vi "main.vi"() -> ()   [LabVIEW 2023]
uses:
  #typedef_States.ctl
  #typedef_DeviceInfo.ctl
panel:
  out "Centrifugation":bool
  in  "Start":bool
  in  "Lid 0pen":bool
  in  "Centrifugation":bool
  out "Lid Open":bool
  out "Blood Cedimentation (OB)":bool
  out "Hormones":bool
  out "Cancer Markers":bool
  out "Blood Cell Count":bool
  out "Centrifugation":bool
  out "Power ON":bool
  in  "Mode":i32(knob)=2 scale=0.0..4.0
  in  "Stop":bool
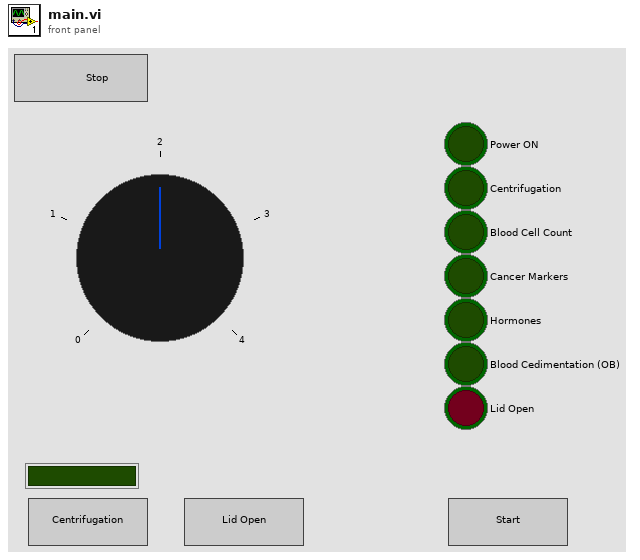
[diagram p1: front panel]
types:
  T1 = typedef "#typedef_States.ctl" = enum16{"Initialize", "Idle", "TestInit", "Test", "LidOpen", "Wait", "TurnOff", "Exit"}
  T2 = enum8{"Enabled", "Disabled", "Disabled and Grayed Out"}
  T3 = typedef "#typedef_DeviceInfo.ctl" = cluster{"Mode":enum16{"Fast Test", "Basic Test", "Power Off", "Full Test", "High Quality Test"}, "Time":cluster{"Centrifugation":i32, "Blood Cell Count":i32, "Cancer Makers":i32, "Hormones":i32, "Blood Cedimentation":i32}, "LidOpenTime":dbl, "Current Time":timestamp, "TestState":i32, "TimeToWait":i32}
  T4 = enum16{"Fast Test", "Basic Test", "Power Off", "Full Test", "High Quality Test"}
  T5 = cluster{"Centrifugation":i32, "Blood Cell Count":i32, "Cancer Makers":i32, "Hormones":i32, "Blood Cedimentation":i32}
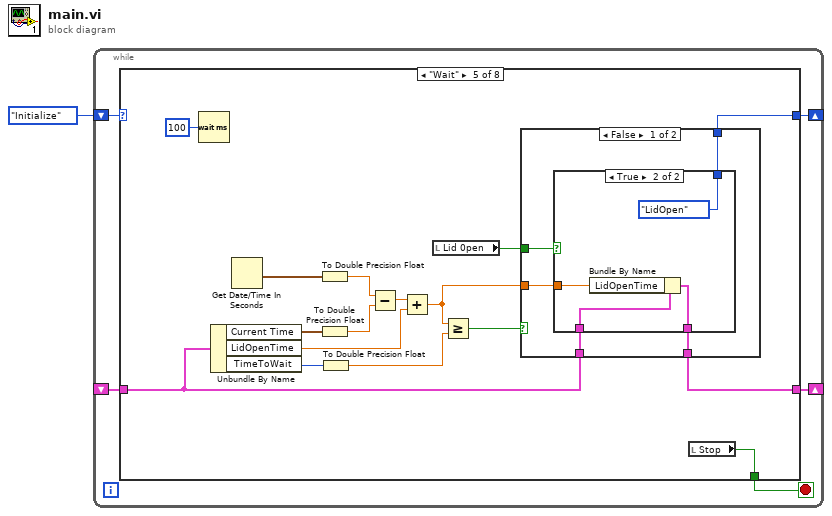
[diagram p0: block diagram]
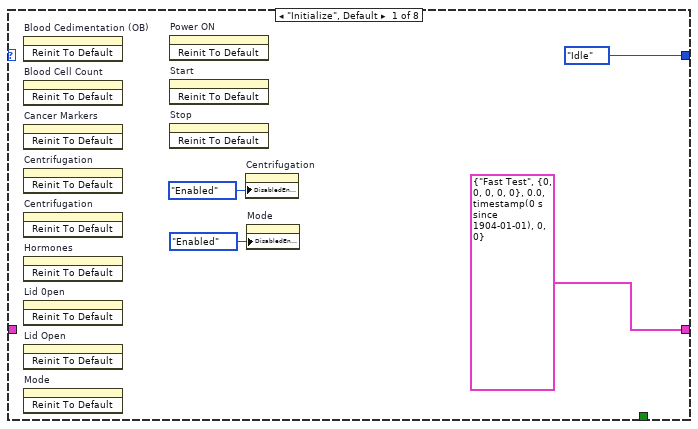
[diagram p2: hidden frame]
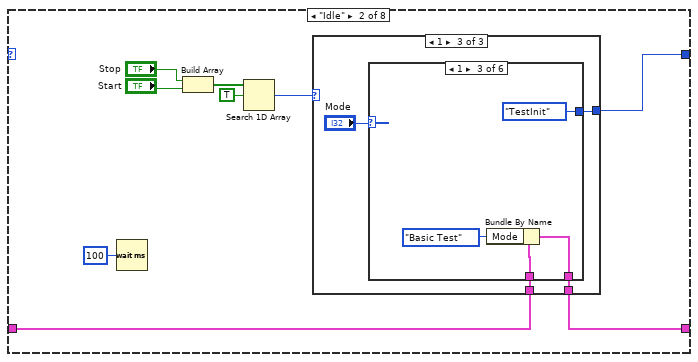
[diagram p3: hidden frame]
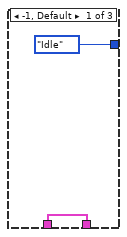
[diagram p4: hidden frame]
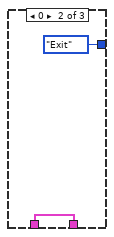
[diagram p5: hidden frame]
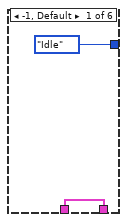
[diagram p6: hidden frame]
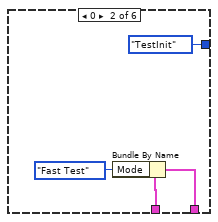
[diagram p7: hidden frame]
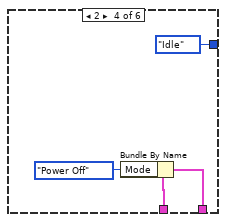
[diagram p8: hidden frame]
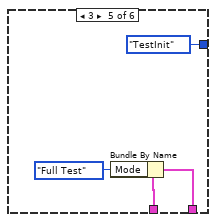
[diagram p9: hidden frame]
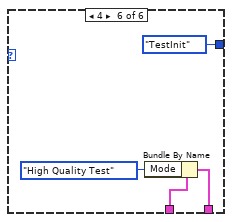
[diagram p10: hidden frame]
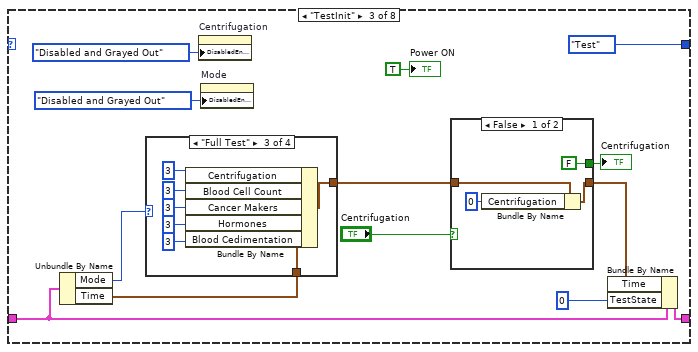
[diagram p11: hidden frame]
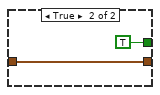
[diagram p12: hidden frame]
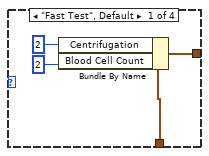
[diagram p13: hidden frame]
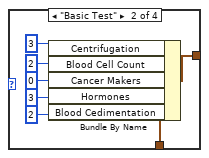
[diagram p14: hidden frame]
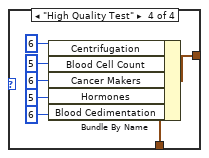
[diagram p15: hidden frame]
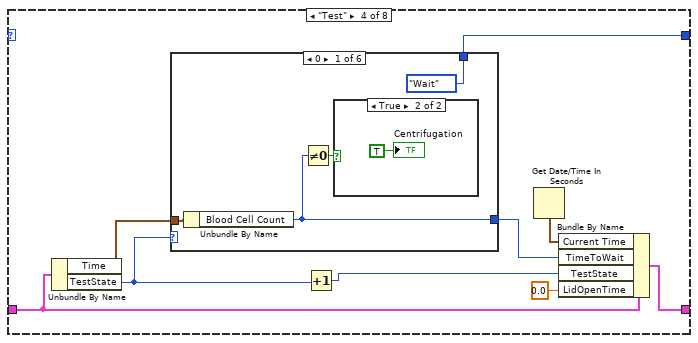
[diagram p16: hidden frame]
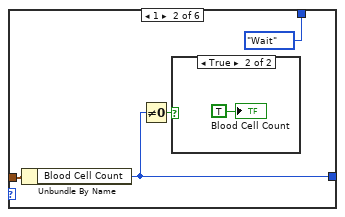
[diagram p18: hidden frame]
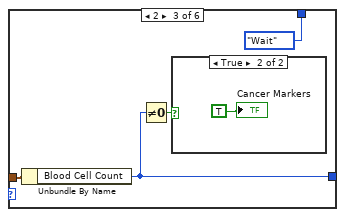
[diagram p20: hidden frame]
diagram:
  n1 = while {
    shift-right: [w5] -> _
    shift-left: #typedef_States."Initialize" ("States") -> [w6]
    shift-right: [w4] -> _
    shift-left: _ -> [w3]
    stop <- w2 stop-if-true
    n2 = case shown="\"Wait\"" w6 {
      tunnel: [#typedef_States."Idle" ("States") w14 #typedef_States."Test" ("States") w98 w133 #typedef_States."Test" ("States") w165 #typedef_States."Exit" ("States")] -> w5
      tunnel: [T3 {"Mode"=enum."Fast Test", "Time"={"Centrifugation"=0, "Blood Cell Count"=0, "Cancer Makers"=0, "Hormones"=0, "Blood Cedimentation"=0}, "LidOpenTime"=0.0, "Current Time"=timestamp(0 s since 1904-01-01), "TestState"=0, "TimeToWait"=0} ("DeviceInfo") w12 w56 w100 w134 w160 w163 w174] -> w4
      tunnel: w3 -> [_ w13 w57 w101 w135 w160 w164 w174]
      tunnel: [_ _ _ _ w140 _ _ TRUE] -> w2
      frame "Initialize", Default {
        n3 = invoke on="Blood Cedimentation (OB)" class="Bool (strict)" method="Reinit To Default"() -> ()  [unwired: 3 in, 3 out]
        n4 = invoke on="Blood Cell Count" class="Bool (strict)" method="Reinit To Default"() -> ()  [unwired: 3 in, 3 out]
        n5 = invoke on="Cancer Markers" class="Bool (strict)" method="Reinit To Default"() -> ()  [unwired: 3 in, 3 out]
        n6 = invoke on="Centrifugation" class="Bool (strict)" method="Reinit To Default"() -> ()  [unwired: 3 in, 3 out]
        n7 = invoke on="Centrifugation" class="Bool (strict)" method="Reinit To Default"() -> ()  [unwired: 3 in, 3 out]
        n8 = invoke on="Hormones" class="Bool (strict)" method="Reinit To Default"() -> ()  [unwired: 3 in, 3 out]
        n9 = invoke on="Lid 0pen" class="Bool (strict)" method="Reinit To Default"() -> ()  [unwired: 3 in, 3 out]
        n10 = invoke on="Lid Open" class="Bool (strict)" method="Reinit To Default"() -> ()  [unwired: 3 in, 3 out]
        n11 = invoke on="Mode" class="Knob (strict)" method="Reinit To Default"() -> ()  [unwired: 3 in, 3 out]
        n12 = invoke on="Power ON" class="Bool (strict)" method="Reinit To Default"() -> ()  [unwired: 3 in, 3 out]
        n13 = invoke on="Start" class="Bool" method="Reinit To Default"() -> ()  [unwired: 3 in, 3 out]
        n14 = invoke on="Stop" class="Bool (strict)" method="Reinit To Default"() -> ()  [unwired: 3 in, 3 out]
        n15 = property on="Centrifugation" class="Bool (strict)"("DisabledEnum"=T2."Enabled" ("Disabled")) -> ()  [unwired: 2 in, 2 out]
        n16 = property on="Mode" class="Knob (strict)"("DisabledEnum"=T2."Enabled" ("Disabled")) -> ()  [unwired: 2 in, 2 out]
      }
      frame "Idle" {
        n17 = Wait (ms)(milliseconds to wait=u32 100) -> ()  [unwired: 1 out]
        n18 = Build Array("Stop", "Start") -> (w19:bool[])
        n19 = Search 1D Array(1D array=w19, element=TRUE) -> (index of element=w15:i32)  [unwired: 1 in]
        n20 = case shown="1" w15 {
          tunnel: [#typedef_States."Idle" ("States") #typedef_States."Exit" ("States") w26] -> w14
          tunnel: w13 -> [w20 w22 w25]
          tunnel: [w20 w22 w24] -> w12
          frame -1, Default {
          }
          frame 0 {
          }
          frame 1 {
            n21 = case shown="1" "Mode" {
              tunnel: [#typedef_States."Idle" ("States") #typedef_States."TestInit" ("States") #typedef_States."TestInit" ("States") #typedef_States."Idle" ("States") #typedef_States."TestInit" ("States") #typedef_States."TestInit" ("States")] -> w26
              tunnel: w25 -> [w28 w32 w36 w40 w44 w48]
              tunnel: [w28 w31 w35 w39 w43 w47] -> w24
              frame -1, Default {
              }
              frame 0 {
                n22 = Bundle By Name(cluster=w32, "Mode"=T4."Fast Test") -> (w31:T3)
              }
              frame 1 {
                n23 = Bundle By Name(cluster=w36, "Mode"=T4."Basic Test") -> (w35:T3)
              }
              frame 2 {
                n24 = Bundle By Name(cluster=w40, "Mode"=T4."Power Off") -> (w39:T3)
              }
              frame 3 {
                n25 = Bundle By Name(cluster=w44, "Mode"=T4."Full Test") -> (w43:T3)
              }
              frame 4 {
                n26 = Bundle By Name(cluster=w48, "Mode"=T4."High Quality Test") -> (w47:T3)
              }
            }
          }
        }
      }
      frame "TestInit" {
        n27 = Unbundle By Name(w57) -> ("Mode"=w61:T4, "Time"=w60:T5)
        n28 = case shown="\"Full Test\"" w61 {
          tunnel: w60 -> [w70 w77 w84 w91]
          tunnel: [w69 w76 w83 w90] -> w58
          frame "Fast Test", Default {
            n29 = Bundle By Name(cluster=w70, "Centrifugation"=2, "Blood Cell Count"=2) -> (w69:T5)
          }
          frame "Basic Test" {
            n30 = Bundle By Name(cluster=w77, "Centrifugation"=3, "Blood Cell Count"=2, "Cancer Makers"=0, "Hormones"=3, "Blood Cedimentation"=2) -> (w76:T5)
          }
          frame "Full Test" {
            n31 = Bundle By Name(cluster=w84, "Centrifugation"=3, "Blood Cell Count"=3, "Cancer Makers"=3, "Hormones"=3, "Blood Cedimentation"=3) -> (w83:T5)
          }
          frame "High Quality Test" {
            n32 = Bundle By Name(cluster=w91, "Centrifugation"=6, "Blood Cell Count"=5, "Cancer Makers"=6, "Hormones"=5, "Blood Cedimentation"=6) -> (w90:T5)
          }
        }
        n33 = property on="Centrifugation" class="Bool (strict)"("DisabledEnum"=T2."Disabled and Grayed Out" ("Disabled")) -> ()  [unwired: 2 in, 2 out]
        n34 = property on="Mode" class="Knob (strict)"("DisabledEnum"=T2."Disabled and Grayed Out" ("Disabled")) -> ()  [unwired: 2 in, 2 out]
        n35 = case shown="False" "Centrifugation" {
          tunnel: w58 -> [w66 w68]
          tunnel: [w64 w68] -> w55
          tunnel: [FALSE ("Centrifugation") TRUE ("Centrifugation")] -> w53
          frame False {
            n36 = Bundle By Name(cluster=w66, "Centrifugation"=0) -> (w64:T5)
          }
          frame True {
          }
        }
        "Centrifugation" <- w53
        n37 = Bundle By Name(cluster=w57, "Time"=w55, "TestState"=0) -> (w56:T3)
        "Power ON" <- TRUE ("Power ON")
      }
      frame "Test" {
        n38 = Unbundle By Name(w101) -> ("Time"=w102:T5, "TestState"=w96:i32)
        n39 = case shown="0" w96 {
          tunnel: w102 -> [w106 w111 w116 w121 w126 _]
          tunnel: [w104 w109 w114 w119 w124 0 ("Blood Cell Count")] -> w97
          tunnel: [#typedef_States."Wait" ("States") #typedef_States."Wait" ("States") #typedef_States."Wait" ("States") #typedef_States."Wait" ("States") #typedef_States."Wait" ("States") #typedef_States."Initialize" ("States")] -> w98
          frame 0 {
            n40 = Unbundle By Name(w106) -> ("Blood Cell Count"=w104:i32)
            n41 = Not Equal To 0?(x=w104) -> (x != 0?=w105:bool)
            n42 = case shown="True" w105 {
              frame False {
              }
              frame True {
                "Centrifugation" <- TRUE ("Blood Cell Count")
              }
            }
          }
          frame 1 {
            n43 = Unbundle By Name(w111) -> ("Blood Cell Count"=w109:i32)
            n44 = Not Equal To 0?(x=w109) -> (x != 0?=w110:bool)
            n45 = case shown="True" w110 {
              frame False {
              }
              frame True {
                "Blood Cell Count" <- TRUE ("Blood Cell Count")
              }
            }
          }
          frame 2 {
            n46 = Unbundle By Name(w116) -> ("Blood Cell Count"=w114:i32)
            n47 = Not Equal To 0?(x=w114) -> (x != 0?=w115:bool)
            n48 = case shown="True" w115 {
              frame False {
              }
              frame True {
                "Cancer Markers" <- TRUE ("Blood Cell Count")
              }
            }
          }
          frame 3 {
            n49 = Unbundle By Name(w121) -> ("Blood Cell Count"=w119:i32)
            n50 = Not Equal To 0?(x=w119) -> (x != 0?=w120:bool)
            n51 = case shown="True" w120 {
              frame False {
              }
              frame True {
                "Hormones" <- TRUE ("Blood Cell Count")
              }
            }
          }
          frame 4 {
            n52 = Unbundle By Name(w126) -> ("Blood Cell Count"=w124:i32)
            n53 = Not Equal To 0?(x=w124) -> (x != 0?=w125:bool)
            n54 = case shown="True" w125 {
              frame False {
              }
              frame True {
                "Blood Cedimentation (OB)" <- TRUE ("Blood Cell Count")
              }
            }
          }
          frame 5, Default {
          }
        }
        n55 = Increment(x=w96) -> (x+1=w95:i32)
        n56 = Get Date/Time In Seconds() -> (seconds since 1Jan1904=w94:timestamp)
        n57 = Bundle By Name(cluster=w101, "Current Time"=w94, "TimeToWait"=w97, "TestState"=w95, "LidOpenTime"=0.0) -> (w100:T3)
      }
      frame "Wait" {
        n58 = Wait (ms)(milliseconds to wait=u32 100) -> ()  [unwired: 1 out]
        n59 = Unbundle By Name(w135) -> ("Current Time"=w144:timestamp, "LidOpenTime"=w138:dbl, "TimeToWait"=w137:i32)
        n60 = Get Date/Time In Seconds() -> (seconds since 1Jan1904=w145:timestamp)
        n61 = To Double Precision Float(number=w145) -> (double precision float=w143:dbl)
        n62 = To Double Precision Float(number=w144) -> (double precision float=w142:dbl)
        n63 = To Double Precision Float(number=w137) -> (double precision float=w136:dbl)
        n64 = Subtract(x=w143, y=w142) -> (x-y=w141:dbl)
        n65 = Add(x=w141, y=w138) -> (x+y=w132:dbl)
        n66 = local read "Lid 0pen"() -> (w130:bool)
        n67 = Greater Or Equal?(x=w132, y=w136) -> (x >= y?=w139:bool)
        n68 = case shown="False" w139 {
          tunnel: w130 -> [w150 _]
          tunnel: [w149 w158] -> w134
          tunnel: w135 -> [w148 w158]
          tunnel: [w147 #typedef_States."TurnOff" ("States")] -> w133
          tunnel: w132 -> [w146 _]
          frame False {
            n69 = case shown="True" w150 {
              tunnel: [w152 w154] -> w149
              tunnel: w148 -> [w152 w155]
              tunnel: [#typedef_States."Wait" ("States") #typedef_States."LidOpen" ("States")] -> w147
              tunnel: w146 -> [_ w153]
              frame False {
              }
              frame True {
                n70 = Bundle By Name(cluster=w155, "LidOpenTime"=w153) -> (w154:T3)
              }
            }
          }
          frame True {
          }
        }
        n71 = local read "Stop"() -> (w140:bool)
      }
      frame "TurnOff" {
        n72 = invoke on="Centrifugation" class="Bool (strict)" method="Reinit To Default"() -> ()  [unwired: 3 in, 3 out]
        n73 = invoke on="Blood Cell Count" class="Bool (strict)" method="Reinit To Default"() -> ()  [unwired: 3 in, 3 out]
        n74 = invoke on="Cancer Markers" class="Bool (strict)" method="Reinit To Default"() -> ()  [unwired: 3 in, 3 out]
        n75 = invoke on="Hormones" class="Bool (strict)" method="Reinit To Default"() -> ()  [unwired: 3 in, 3 out]
        n76 = invoke on="Blood Cedimentation (OB)" class="Bool (strict)" method="Reinit To Default"() -> ()  [unwired: 3 in, 3 out]
      }
      frame "LidOpen" {
        n77 = Wait (ms)(milliseconds to wait=u32 100) -> ()  [unwired: 1 out]
        n78 = case shown="False" "Lid 0pen" {
          tunnel: [#typedef_States."Wait" ("States") #typedef_States."LidOpen" ("States")] -> w165
          tunnel: [w167 w171] -> w163
          tunnel: w164 -> [w169 w171]
          frame False {
            n79 = Get Date/Time In Seconds() -> (seconds since 1Jan1904=w168:timestamp)
            n80 = Bundle By Name(cluster=w169, "Current Time"=w168) -> (w167:T3)
            n81 = invoke on="Lid Open" class="Bool (strict)" method="Reinit To Default"() -> ()  [unwired: 3 in, 3 out]
          }
          frame True {
          }
        }
        "Lid Open" <- TRUE ("Lid Open")
      }
      frame "Exit" {
      }
    }
  }
